vi "Supply_ComplianceCheck.vi"(8 "error in (no error)":errorcluster, 11 "KE2657A in":refnum<class "KE2657A.lvclass">) -> (0 "error out":errorcluster, 1 "Status string":string, 2 "Compliance exceeded?":bool, 3 "KE2657A out":refnum<class "KE2657A.lvclass">)   [LabVIEW 2018, in "KE2657A.lvclass"]
uses:
  KE2657A.lvclass
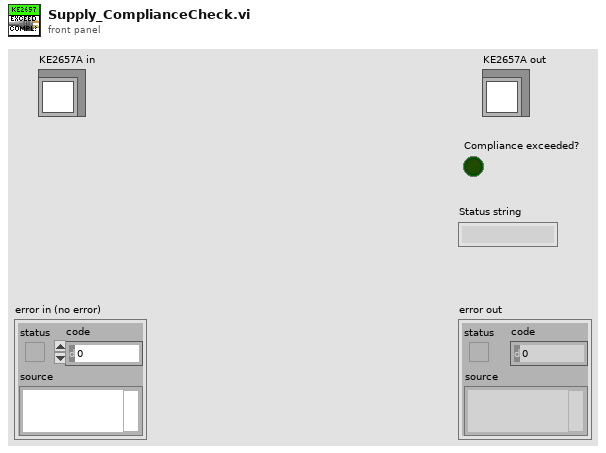
[diagram p1: front panel]
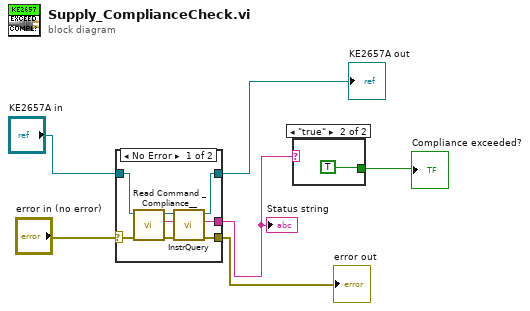
[diagram p0: block diagram]
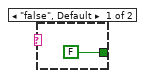
[diagram p2: hidden frame]
diagram:
  n1 = case shown="No Error" "error in (no error)" {
    selector: "error in (no error)" -> [w7 w15]
    tunnel: [w14 w15] -> w4
    tunnel: [w13 w16] -> w3
    tunnel: "KE2657A in" -> [w9 w16]
    tunnel: [w8 _] -> w2
    frame No Error {
      n2 = call-dynamic "Read Command _Compliance__.vi"("error in (no error)"=w7, "SupplyControl in"=w9) -> ("error out"=w12:errorcluster, "Command \"Compliance?\""=w11:string, "SupplyControl out"=w10:refnum<class "KE2657A.lvclass">)  [unwired: 7 in]
      n3 = call-dynamic "InstrQuery.vi"("error in (no error)"=w12, "Command string"=w11, "InstControl in"=w10) -> ("error out"=w14:errorcluster, "Instrument response"=w8:string, "InstControl out"=w13:refnum<class "KE2657A.lvclass">)  [unwired: 6 in]
    }
    frame Error {
    }
  }
  "KE2657A out" <- w3
  "error out" <- w4
  "Status string" <- w2
  n4 = case shown="\"true\"" w2 {
    tunnel: [FALSE TRUE] -> w1
    frame "false", Default {
    }
    frame "true" {
    }
  }
  "Compliance exceeded?" <- w1
